vi "PRIME Detector Test Program.vi"() -> ()   [LabVIEW 2021, in "PRIME Detector.lvclass"]
uses:
  PRIME Detector.lvclass
  RIMAS Detector Server Config.ctl
  PRIME Detector cluster Status.ctl
  <vilib>/JDP Science/JSONtext/JSONtext.lvlib
panel:
  out "Status Response":string
  out "Status":T1
  out "error out":errorcluster
  in  "Detector Computer":T2={"Machine"="192.168.121.11", "Password"="rSL!nux23456", "FITS File Path"="", "Port"=44444, "Header Path"="", "Name"=""}
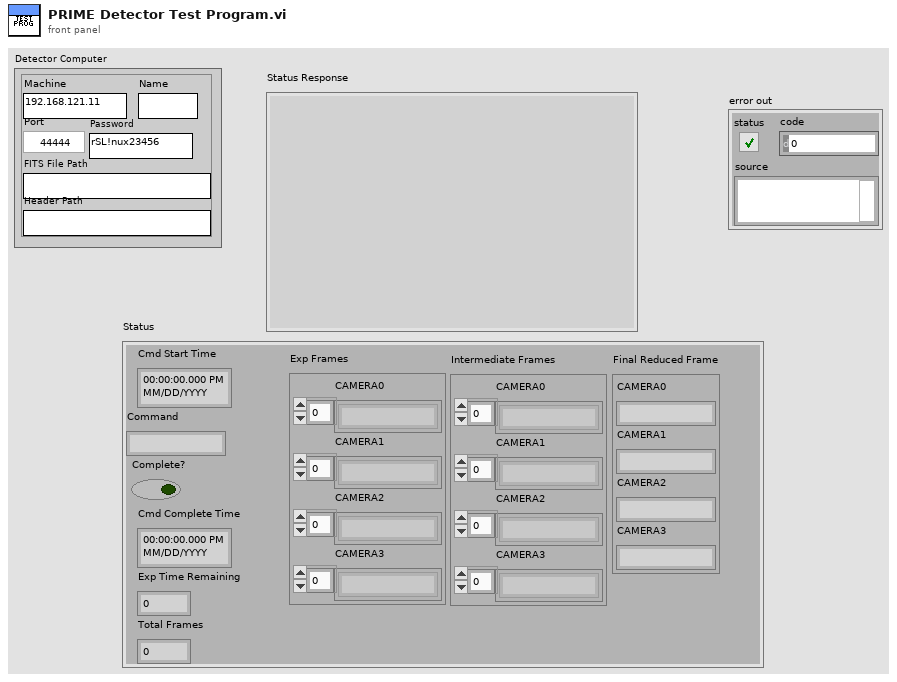
[diagram p1: front panel]
types:
  T1 = typedef "PRIME Detector cluster Status.ctl" = cluster{"Cmd Start Time":timestamp, "Command":string, "Complete?":bool, "Cmd Complete Time":timestamp, "Exp Time Remaining":dbl, "Total Frames":i32, "Exp Frames":cluster{"CAMERA0":string[], "CAMERA1":string[], "CAMERA2":string[], "CAMERA3":string[]}, "Intermediate Frames":cluster{"CAMERA0":string[], "CAMERA1":string[], "CAMERA2":string[], "CAMERA3":string[]}, "Final Reduced Frame":cluster{"CAMERA0":string, "CAMERA1":string, "CAMERA2":string, "CAMERA3":string}}
  T2 = typedef "RIMAS Detector Server Config.ctl" = cluster{"Machine":string, "Password":string, "FITS File Path":string, "Port":u16, "Header Path":string, "Name":string}
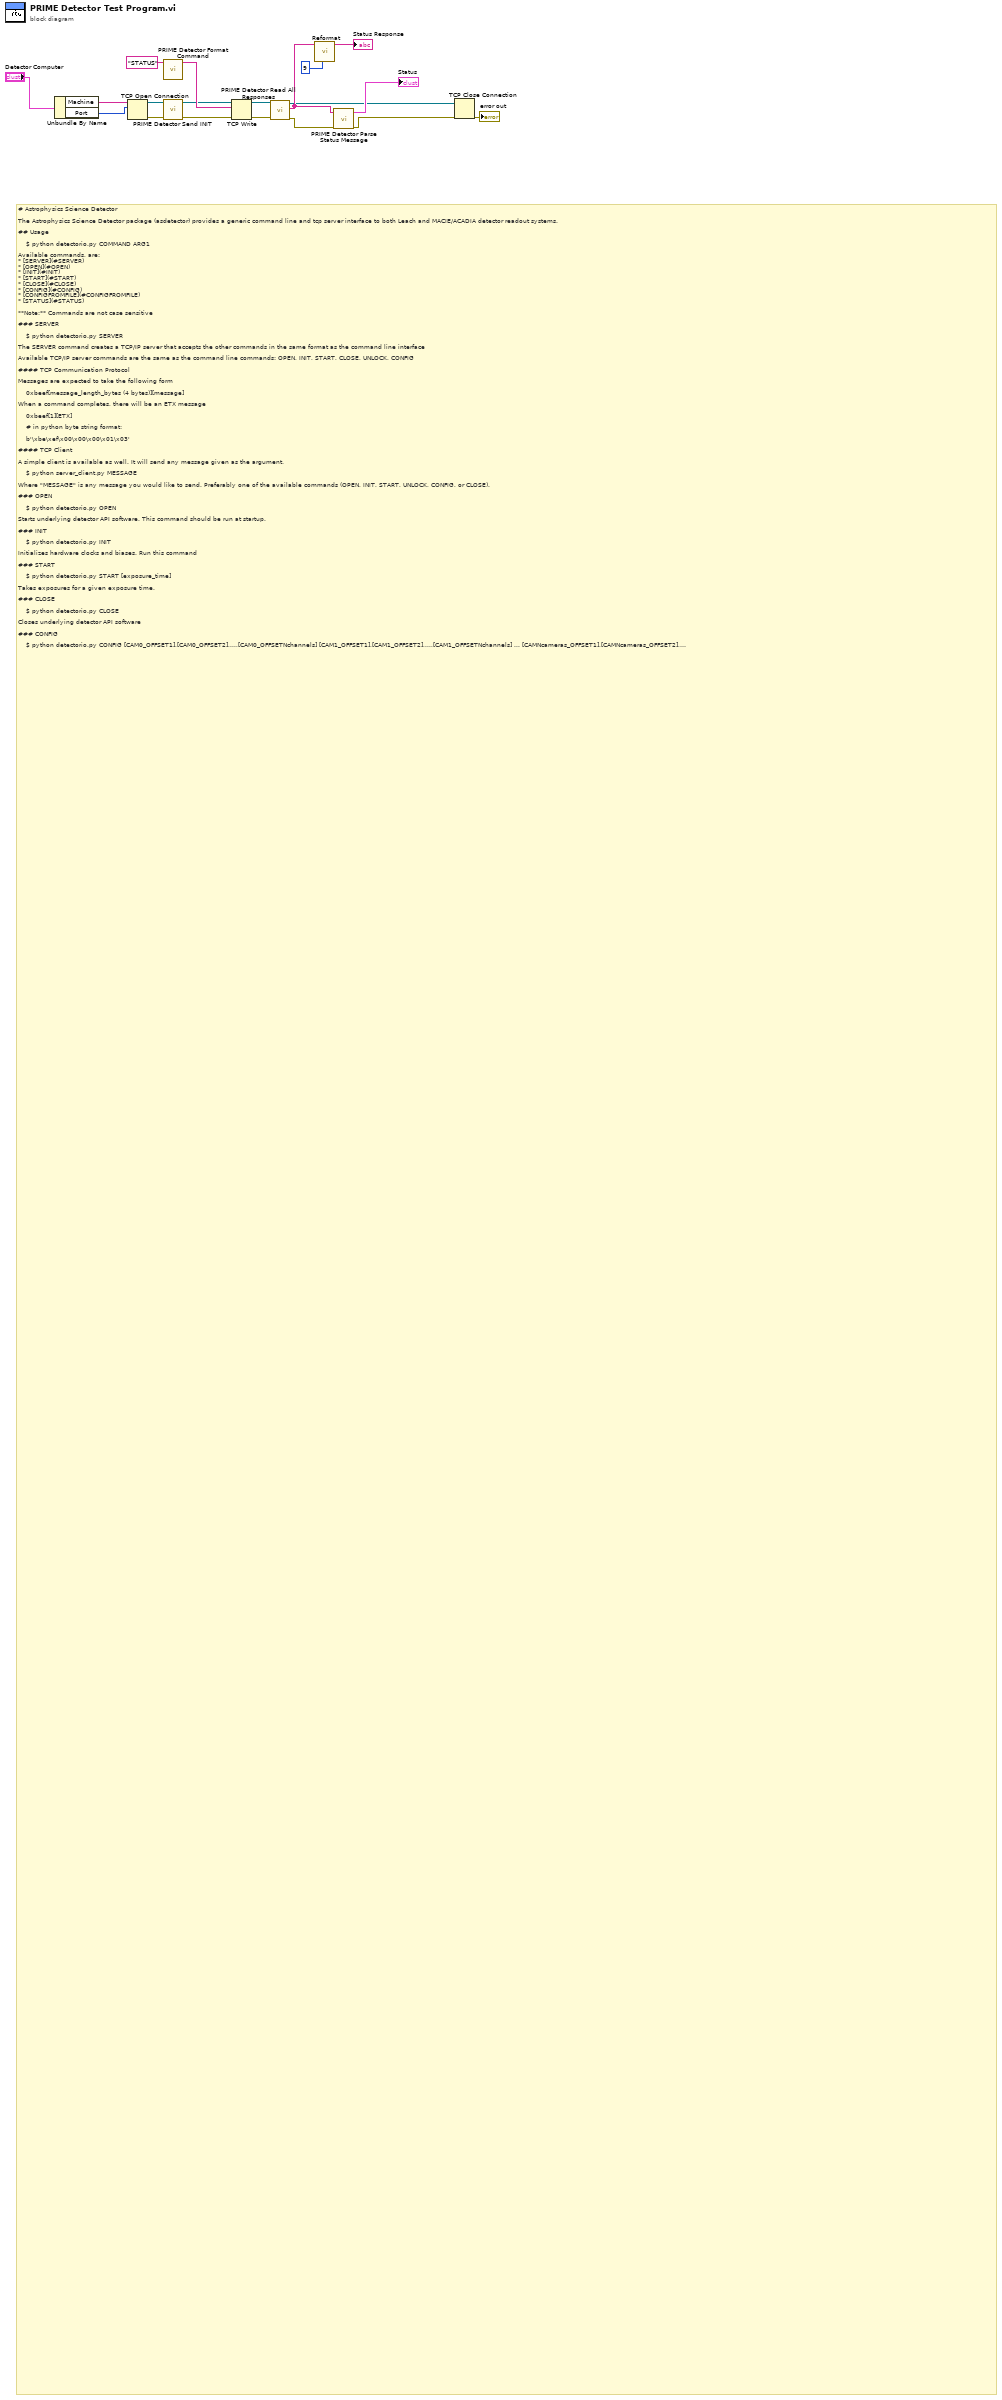
[diagram p0: block diagram]
diagram:
  # "# Astrophysics Science Detector\n\nThe Astrophysics Science Detector package (asdetector) provides a generic command line and tcp server interface to both Leach and MACIE/ACADIA detector readout systems.\n\n## Usage\n    \n    $ python detectorio.py COMMAND ARG1\n\nAvailable commands, are:\n* [SERVER](#SERVER)\n* [OPEN](#OPEN)\n* [INIT](#INIT)\n* [START](#START)\n* [CLOSE](#CLOSE)\n* [CONFIG](#CONFIG)\n* [CONFIGFROMFILE](#CONFIGFROMFILE)\n* [STATUS](#STATUS)\n\n**Note:** Commands are not case sensitive\n\n### SERVER\n\n    $ python detectorio.py SERVER\n    \nThe SERVER command creates a TCP/IP server that accepts the other commands in the same format as the command line interface\n\nAvailable TCP/IP server commands are the same as the command line commands: OPEN, INIT, START, CLOSE, UNLOCK, CONFIG\n\n#### TCP Communication Protocol\n\nMessages are expected to take the following form\n\n    0xbeef[message_length_bytes (4 bytes)][message]\n\nWhen a command completes, there will be an ETX message\n\n    0xbeef[1][ETX]\n    \n    # in python byte string format:\n    \n    b'\\xbe\\xef\\x00\\x00\\x00\\x01\\x03'\n\n#### TCP Client\n\nA simple client is available as well. It will send any message given as the argument.\n\n    $ python server_client.py MESSAGE\n\nWhere \"MESSAGE\" is any message you would like to send. Preferably one of the available commands (OPEN, INIT, START, UNLOCK, CONFIG, or CLOSE).\n\n### OPEN\n\n    $ python detectorio.py OPEN\n\nStarts underlying detector API software. This command should be run at startup.\n\n### INIT\n\n    $ python detectorio.py INIT\n    \nInitializes hardware clocks and biases. Run this command \n\n### START\n\n    $ python detectorio.py START [exposure_time]\n\nTakes exposures for a given exposure time.\n\n### CLOSE\n\n    $ python detectorio.py CLOSE \n    \nCloses underlying detector API software\n\n### CONFIG\n\n    $ python detectorio.py CONFIG [CAM0_OFFSET1],[CAM0_OFFSET2],...,[CAM0_OFFSETNchannels] [CAM1_OFFSET1],[CAM1_OFFSET2],...,[CAM1_OFFSETNchannels] ... [CAMNcameras_OFFSET1],[CAMNcameras_OFFSET2],...,[CAMNcameras_OFFSETNchannels]\n\nSets the individual channel offsets based on hex code between 000 and FFF. \n\nExample:\n\n    $ python detectorio.py CONFIG 360,361,365,36F,370,35B,361,365,36F,370,35B,361,365,36F,370,35B,361,365,36F,370,35B,361,365,36F,370,35B,361,365,36F,370,35B,3FF 360,361,365,36F,370,35B,361,365,36F,370,35B,361,365,36F,370,35B,361,365,36F,370,35B,361,365,36F,370,35B,361,365,36F,370,35B,3FF\n\n### CONFIGFROMFILE\n\n    $ python detectorio.py CONFIGFROMFILE [offsets_file]\n\nSets the individual channel offsets based on hex code between 000 and FFF using data from data in a space separated dat file.\n\nExample that replicates the CONFIG example:\n\n    $ python detectorio.py CONFIGFROMFILE /path/to/offsets.dat\n\nWhere offsets.dat contains the follwing text:\n\n    360 360\n    361 361\n    365 365\n    36f 36f\n    370 370\n    35b 35b\n    361 361\n    365 365\n    36f 36f\n    370 370\n    35b 35b\n    361 361\n    365 365\n    36f 36f\n    370 370\n    35b 35b\n    361 361\n    365 365\n    36f 36f\n    370 370\n    35b 35b\n    361 361\n    365 365\n    36f 36f\n    370 370\n    35b 35b\n    361 361\n    365 365\n    36f 36f\n    370 370\n    35b 35b\n    3ff 3ff\n\n### STATUS\n\n    $ python detectorio.py STATUS\n    \nReturns the JSON string contained in the JSON status file\n\n#### JSON Status File\n\nThe JSON Status file, status/status.json, has the following format:\n\n    {\n      \"CommandStartTime\": \"\",\n      \"CurrentCommand\": \"\",\n      \"CommandComplete\": false,\n      \"CommandCompleteTime\": \"\",\n      \"ExposureTimeRemaining\": -9999.9,\n      \"TotalFrameCount\": -9999,\n      \"ExposureFrames\": {\n        \"CAMERA0\": [],\n        \"CAMERA1\": [],\n        \"CAMERA2\": [],\n        \"CAMERA3\": []\n      },\n      \"IntermediateReducedFrames\": {\n        \"CAMERA0\": [],\n        \"CAMERA1\": [],\n        \"CAMERA2\": [],\n        \"CAMERA3\": []\n      },\n      \"FinalReducedFrame\": {\n        \"CAMERA0\": \"\",\n        \"CAMERA1\": \"\",\n        \"CAMERA2\": \"\",\n        \"CAMERA3\": \"\"\n      }\n    }\n\n### Field definitions\n\n* _CommandStartTime_ - Time when command was made\n* _CurrentCommand_ - Command being executed\n* _CommandComplete_ - Flags whether a command has completed\n* _CommandCompleteTime_ - Time command was completed. Blank until command is complete\n* _ExposureTimeRemaining_ - Time remaining in current exposure. Particular to START command\n* _TotalFrameCount_ - Total raw frames for an exposure. Particular to START command\n* _ExposureFrames_ - Dictionary containing a list for each camera with the absolute paths to the raw fits files for an exposure in chronological order. Particular to START command\n* _IntermediateReducedFrames_ - Dictionary containing a list for each camera with the absolute paths to the bias subtracted fits files for an exposure in chronological order. These lightly processed frames are typically more useful for an observer. Particular to START command\n* _FinalReducedFrame_ - Dictionary containing single reduced frame an exposure for each camera. This appears at the end of an exposure, and is the file the observer will take home with them. Particular to START command\n\n## Installation\n\n1) Install underlying API software, MACIE library or ARC API.\n2) If not installed already, install python. I recommend [miniconda](https://docs.conda.io/en/latest/miniconda.html)\n3) Install the required packages\n\n    a) If you are using conda:\n        \n       $ conda install six astropy numpy matplotlib\n        \n    b) If you are using pip:\n        \n       $ pip install six astropy numpy matplotlib\n4) Clone the repository:\n\n       $ git clone https://sed-gitlab.gsfc.nasa.gov/jdurbak/asdetector\n    \n5) Configure [settings](#Settings) if you want want to change default settings.\n\n6) Run the interface\n\n       $ python detectorio.py --help\n\n## TCP Client\n\nThis module comes with a TCP client if you want to interact with the TCP server started by the `python detectorio.py SERVER` command.\n\nUsage:\n\n    $ python server_client.py [COMMAND] [ARG1] [ARG2]\n\nExample:\n\n    $ python server_client.py START 300\n\n## Settings\n\nDetector Readout settings should appear in the main folder in a file called settings.json. Templates can be found for \n[Leach](https://sed-gitlab.gsfc.nasa.gov/jdurbak/asdetector/-/blob/master/settings.json.leachtemplate) and\n[MACIE](https://sed-gitlab.gsfc.nasa.gov/jdurbak/asdetector/-/blob/master/settings.json.macietemplate) readout systems.\n\nIf a key is missing in the settings.json file, or if there is no settings.json file, the default will be used.\n\nDefault settings dictionary:\n\n    DEFAULT_SETTINGS = {\n        'READOUTHARDWARE': 'MACIE',\n        'NUMBEROFCAMERAS': 4,\n        'NUMBEROFREADOUTCHANNELS': 32\n    }"
  n1 = Unbundle By Name("Detector Computer") -> ("Machine"=w18:string, "Port"=w17:u16)
  n2 = TCP Open Connection(address=w18, remote port or service name=w17) -> (connection ID=w6:refnum<k5>, error out=w4:errorcluster)  [unwired: 3 in]
  n3 = call "PRIME Detector Format Command.vi"("Command"="STATUS") -> ("TCP String"=w15:string)  [unwired: 10 in]
  n4 = call "PRIME Detector Send INIT.vi"("error in (no error)"=w4, "connection ID"=w6) -> ("error out"=w3:errorcluster, "connection ID out"=w5:refnum<k5>)  [unwired: 8 in]
  n5 = TCP Write(connection ID=w5, data in=w15, error in (no error)=w3) -> (connection ID out=w13:refnum<k5>, error out=w12:errorcluster)  [unwired: 1 in, 1 out]
  n6 = call "PRIME Detector Read All Responses.vi"("error in"=w12, "connection ID"=w13) -> ("error out"=w10:errorcluster, "Status Response"=w7:string, "connection ID out"=w2:refnum<k5>)  [unwired: 6 in, 1 out]
  n7 = call <vilib>:"Reformat.vi"("Pretty Print Levels"=9, "JSON"=w7) -> ("<JSON>"=→"Status Response":string)  [unwired: 6 in, 3 out]
  n8 = call "PRIME Detector Parse Status Message.vi"("error in (no error)"=w10, "JSON"=w7) -> ("error out"=w1:errorcluster, "status"=→"Status":T1)  [unwired: 8 in]
  n9 = TCP Close Connection(connection ID=w2, error in (no error)=w1) -> (error out=→"error out":errorcluster)  [unwired: 1 in, 1 out]
